vi "LibXML_GetValues.vi"(6 "Node-Type":enum16{"Attribute", "Element"}(ring), 8 "error in":errorcluster, 9 "Name":string, 10 "Root-path (xpath)":string, 11 "doc":u32) -> (0 "error out":errorcluster, 1 "First Value":string, 2 "Values":string[](array[string]), 3 "doc copy out":u32, 4 "#ofNodes":u32)   [LabVIEW 2019, in "Tools.lvlib" / "LibXML.lvlib"]
doc: "This vi searches values of attributes or elements in the given rootpath. If there ar more elements in the rootpath with the same name all values are found and put in the values-array. When only one value is expected (like in attributes) one can use the first value output.\nThe syntax for the rootpath is the XPath-syntax\nIf we want to find the values of the attribute\"axis\" of all ReadAxis elements under the ReadMethod element of the Datachannel with attribute name-id =\"Scan-data the root-path will be\n.//DataChannel[@name-id =\"Scan-data \"]/ReadMethod//ReadAxis\n while the name input should be axis, and the node type should be Attribute."
uses:
  LibXML.lvlib
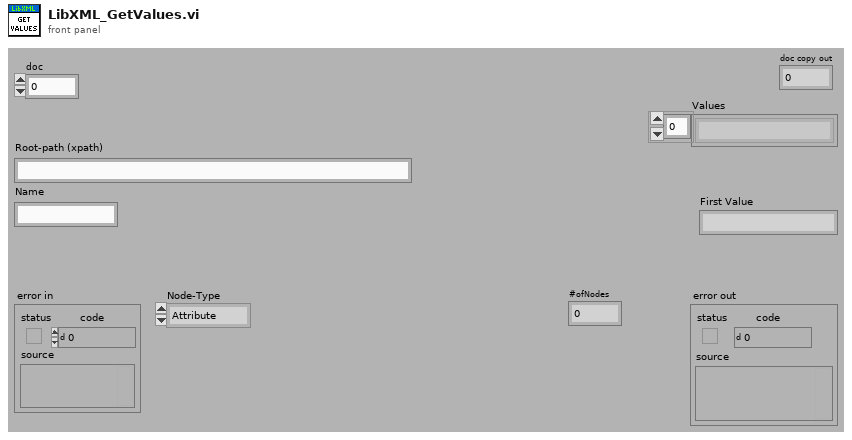
[diagram p1: front panel]
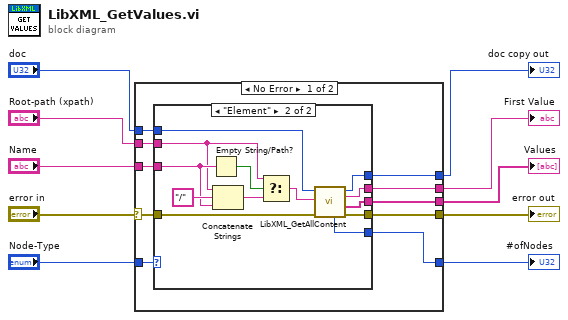
[diagram p0: block diagram]
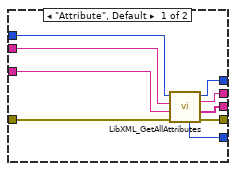
[diagram p2: hidden frame]
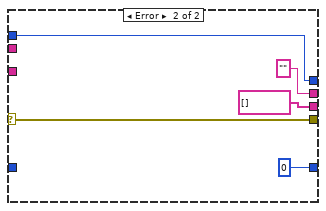
[diagram p3: hidden frame]
diagram:
  n1 = case shown="No Error" "error in" {
    selector: "error in" -> [w20 w46]
    tunnel: [w16 string[] []] -> w7
    tunnel: [w18 w46] -> w10
    tunnel: "doc" -> [w19 w43]
    tunnel: [w17 ""] -> w4
    tunnel: [w15 u32 0 ("#ofNodes")] -> w6
    tunnel: [w14 w43] -> w5
    tunnel: "Node-Type" -> [w13 _]
    tunnel: "Root-path (xpath)" -> [w12 _]
    tunnel: "Name" -> [w11 _]
    frame No Error {
      n2 = case shown="\"Element\"" w13 {
        tunnel: w12 -> [w26 w33]
        tunnel: w11 -> [w25 w34]
        tunnel: w20 -> [w29 w41]
        tunnel: w19 -> [w27 w40]
        tunnel: [w23 w39] -> w14
        tunnel: [w22 w38] -> w17
        tunnel: [w21 w37] -> w16
        tunnel: [w28 w36] -> w18
        tunnel: [w24 w35] -> w15
        frame "Attribute", Default {
          n3 = call "LibXML_GetAllAttributes.vi"("error in"=w29, "attr. name"=w25, "xpathexpr (root)"=w26, "doc"=w27) -> ("error out"=w28:errorcluster, "value list"=w21:string[], "value"=w22:string, "doc copy out"=w23:u32, "#ofNodes"=w24:u32)  [unwired: 3 in]
        }
        frame "Element" {
          n4 = Empty String/Path?(string/path=w34) -> (empty?=w32:bool)
          n5 = Concatenate Strings(w33, "/" ("string"), w34) -> (w31:string)
          n6 = Select(t=w33, s=w32, f=w31) -> (s? t:f=w30:string)
          n7 = call "LibXML_GetAllContent.vi"("error in"=w41, "xpathexpr"=w30, "doc in"=w40) -> ("error out"=w36:errorcluster, "content list"=w37:string[], "content"=w38:string, "doc copy out"=w39:u32, "#ofNodes"=w35:u32)  [unwired: 4 in]
        }
      }
    }
    frame Error {
    }
  }
  "Values" <- w7
  "error out" <- w10
  "First Value" <- w4
  "#ofNodes" <- w6
  "doc copy out" <- w5
